vi "MakeRoom.vi"(7 "RoomID":T1, 8 "error in (no error)":errorcluster, 10 "RoomNumber":i32, 11 "MazeGame":refnum<class "MazeGame.lvclass">) -> (0 "error out":errorcluster, 2 "Room":refnum<class "Room.lvclass">, 3 "MazeGame":refnum<class "MazeGame.lvclass">)   [LabVIEW 2020, in "FactoryMethod.lvlib" / "ParameterizedFactoryMethod.lvlib" / "MazeGame.lvclass"]
uses:
  MazeGame.lvclass
  GoFcommonClasses/ConcreteMazeSite/Room/Room.lvclass
  TypeDef/RoomID.ctl
  GoFcommonClasses/ConcreteMazeSite/RoomWithBomb/RoomWithBomb.lvclass
  E:/Francesco/GitHub/Design-Patterns-GoF_-_NI-LV/Creational/GoFcommonClasses/ConcreteMazeSite/Room/Room.lvclass
  GoFcommonClasses/ConcreteMazeSite/EnchantedRoom/EnchantedRoom.lvclass
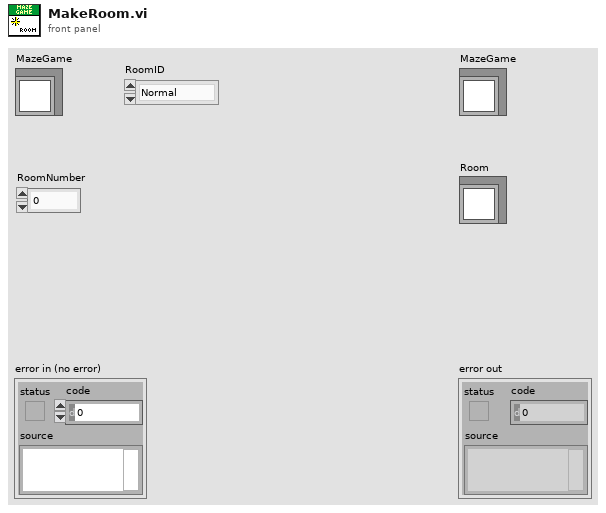
[diagram p1: front panel]
types:
  T1 = typedef "FactoryMethod.lvlib/ParameterizedFactoryMethod.lvlib/MazeGame.lvclass/RoomID.ctl" = enum16{"Normal", "Bombed", "Enchanted"}
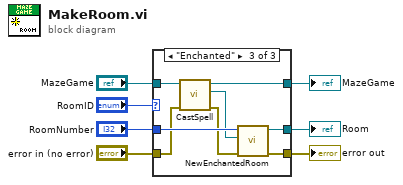
[diagram p0: block diagram]
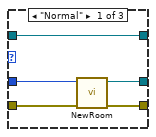
[diagram p2: hidden frame]
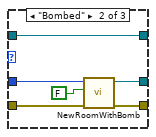
[diagram p3: hidden frame]
diagram:
  n1 = case shown="\"Enchanted\"" "RoomID" {
    tunnel: [w12 w17 w24] -> w7
    tunnel: "RoomNumber" -> [w11 w15 w26]
    tunnel: "error in (no error)" -> [w10 w16 w19]
    tunnel: [w9 w18 w25] -> w4
    tunnel: "MazeGame" -> [w8 w13 w21]
    tunnel: [w8 w13 w20] -> w1
    frame "Normal" {
      n2 = call "NewRoom.vi"("error in (no error)"=w10, "RoomNumber"=w11) -> ("error out"=w9:errorcluster, "Room"=w12:refnum<class "Room.lvclass">)  [unwired: 8 in]
    }
    frame "Bombed" {
      n3 = call "NewRoomWithBomb.vi"("error in (no error)"=w16, "Bombed"=FALSE, "RoomNumber"=w15) -> ("error out"=w18:errorcluster, "RoomWithBomb"=w17:refnum<class "RoomWithBomb.lvclass">)  [unwired: 7 in]
    }
    frame "Enchanted" {
      n4 = call "CastSpell.vi"("error in (no error)"=w19, "MazeGame"=w21) -> ("error out"=w23:errorcluster, "Spell"=w22:refnum<class "Spell.lvclass">, "MazeGame"=w20:refnum<class "MazeGame.lvclass">)  [unwired: 7 in]
      n5 = call "NewEnchantedRoom.vi"("error in (no error)"=w23, "Spell"=w22, "RoomNumber"=w26) -> ("error out"=w25:errorcluster, "EnchantedRoom"=w24:refnum<class "EnchantedRoom.lvclass">)  [unwired: 7 in]
    }
  }
  "error out" <- w4
  "MazeGame" <- w1
  "Room" <- w7
